vi "Read Transition Profile.vi"(8 "error in (no error)":errorcluster, 11 "signal configuration":refnum<class "SV Signal.lvclass">) -> (0 "error out":errorcluster, 2 "transition profile":enum16{"Immediate", "Next optimum", "Ramp"}(ring)=enum."Next optimum", 3 "signal configuration":refnum<class "SV Signal.lvclass">)   [LabVIEW 2017, in "SV Signal.lvclass"]
uses:
  <vilib>/addons/_NISVFA/_Generation/Signal Generation/SV Signal/SV Signal.lvclass
  <vilib>/addons/_NISVFA/_Generation/Signal Generation/SV Signal/SV Signal.lvclass/SV Signal.ctl
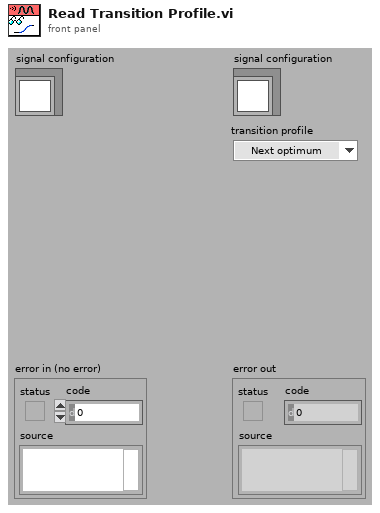
[diagram p1: front panel]
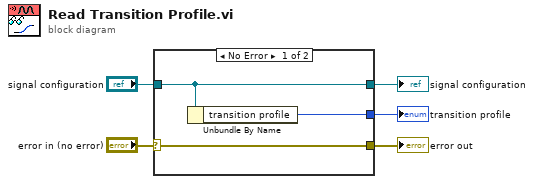
[diagram p0: block diagram]
diagram:
  n1 = case shown="No Error" "error in (no error)" {
    selector: "error in (no error)" -> [w8 w9]
    tunnel: [w8 w9] -> w4
    tunnel: [w7 w10] -> w2
    tunnel: "signal configuration" -> [w7 w10]
    tunnel: [w6 _] -> w1
    frame No Error {
      n2 = Unbundle By Name(w7) -> ("transition profile"=w6:enum16{"Immediate", "Next optimum", "Ramp"})
    }
    frame Error {
    }
  }
  "error out" <- w4
  "signal configuration" <- w2
  "transition profile" <- w1
